vi "Form Message Log Text.vi"(9 "Data String Input":string, 10 "Module Action":string, 11 "Ack Requested":bool) -> (3 "String to Write":string)   [LabVIEW 2015, in "Generic Module Library.lvlib" / "Template G_Module.lvlib"]
uses:
  Template G_Module.lvlib
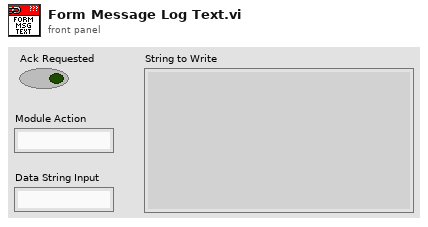
[diagram p1: front panel]
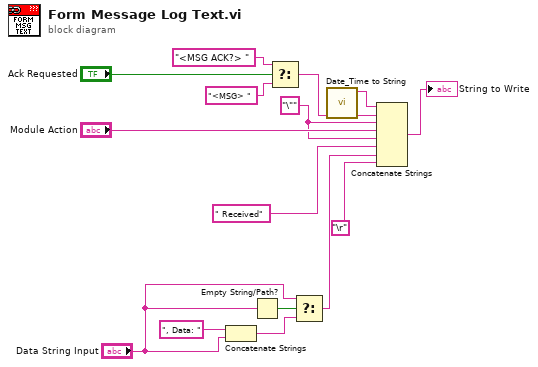
[diagram p0: block diagram]
diagram:
  w1 = "\"" ("string")
  n1 = Concatenate Strings(", Data: " ("string"), "Data String Input") -> (w14:string)
  n2 = Empty String/Path?(string/path="Data String Input") -> (empty?=w12:bool)
  n3 = Select(t="<MSG ACK?> ", s="Ack Requested", f="<MSG> ") -> (s? t:f=w7:string)
  n4 = Select(t="Data String Input", s=w12, f=w14) -> (s? t:f=w4:string)
  n5 = call "Date_Time to String.vi"() -> ("date/time string"=w9:string)  [unwired: 11 in]
  n6 = Concatenate Strings(w9, w7, w1, "Module Action", w1, " Received" ("string"), w4, "\r") -> (→"String to Write":string)
